vi "GPS Satelites.vi"() -> ()   [LabVIEW 2016]
panel:
  in  "Satelites":i16
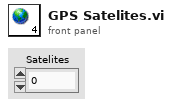
[diagram p1: front panel]
diagram:
